vi "clFileReader_getNewReader.vi"(9 "DataLenght":i32=-1, 10 "HiddenOffset":u32, 11 "clFileReader.lvclass":refnum<class "clFileReader.lvclass">) -> (2 "New clFileReader":refnum<class "clFileReader.lvclass">)   [LabVIEW 2011, in "vi_lib.lvlib" / "clFileReader.lvclass"]
uses:
  clFileReader.lvclass
  clFileReader.lvclass/clFileReader.ctl
  clFile/clFile.lvclass
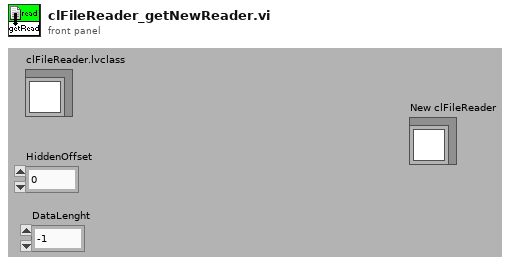
[diagram p1: front panel]
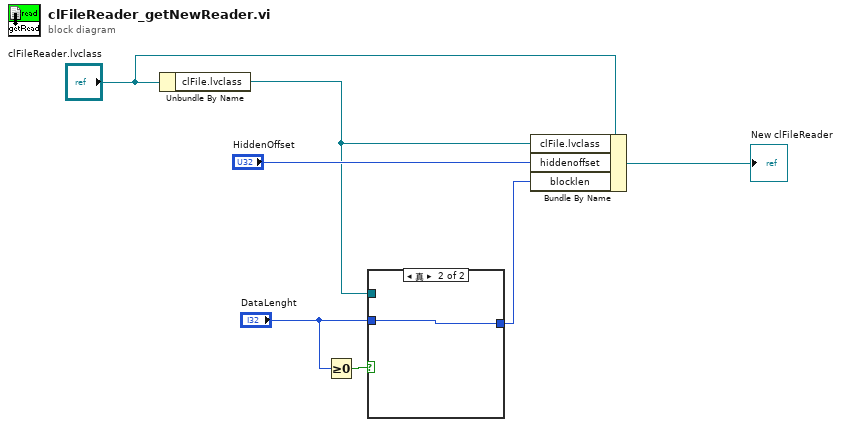
[diagram p0: block diagram]
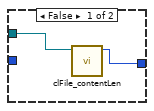
[diagram p2: hidden frame]
diagram:
  n1 = Unbundle By Name("clFileReader.lvclass") -> ("clFile.lvclass"=w2:refnum<class "clFile.lvclass">)
  n2 = Greater Or Equal To 0?(x="DataLenght") -> (x >= 0?=w6:bool)
  n3 = case shown="真" w6 {
    tunnel: "DataLenght" -> [_ w10]
    tunnel: [w9 w10] -> w4
    tunnel: w2 -> [w8 _]
    frame False {
      n4 = call "clFile_contentLen.vi"("clFile.lvclass"=w8) -> ("length"=w9:u32)  [unwired: 10 out]
    }
    frame True {
    }
  }
  n5 = Bundle By Name(cluster="clFileReader.lvclass", "clFile.lvclass"=w2, "hiddenoffset"="HiddenOffset", "blocklen"=w4) -> (→"New clFileReader":refnum<class "clFileReader.lvclass">)
